vi "trial 2.vi"() -> ()   [LabVIEW 2013]
panel:
  in  "Contours":T1(array[cluster])
  in  "Global Rectangle":i32[](array[numeric])
  in  "ROI Descriptor":T2 {"Contours"."Type" items=["No Selection", "Point", "Line", "Rectangle", "Oval", "Polygon", "Freehand Region", "Annulus", "Unused2", "Unused3", "Broken Line", "Freehand Line", "Rotated Rectangle"]}
  in  "Play":bool
  in  "stop":bool
  in  "Pause":bool
  out "Image 3":T3(plugin-control)
  in  "AVI File Path":path
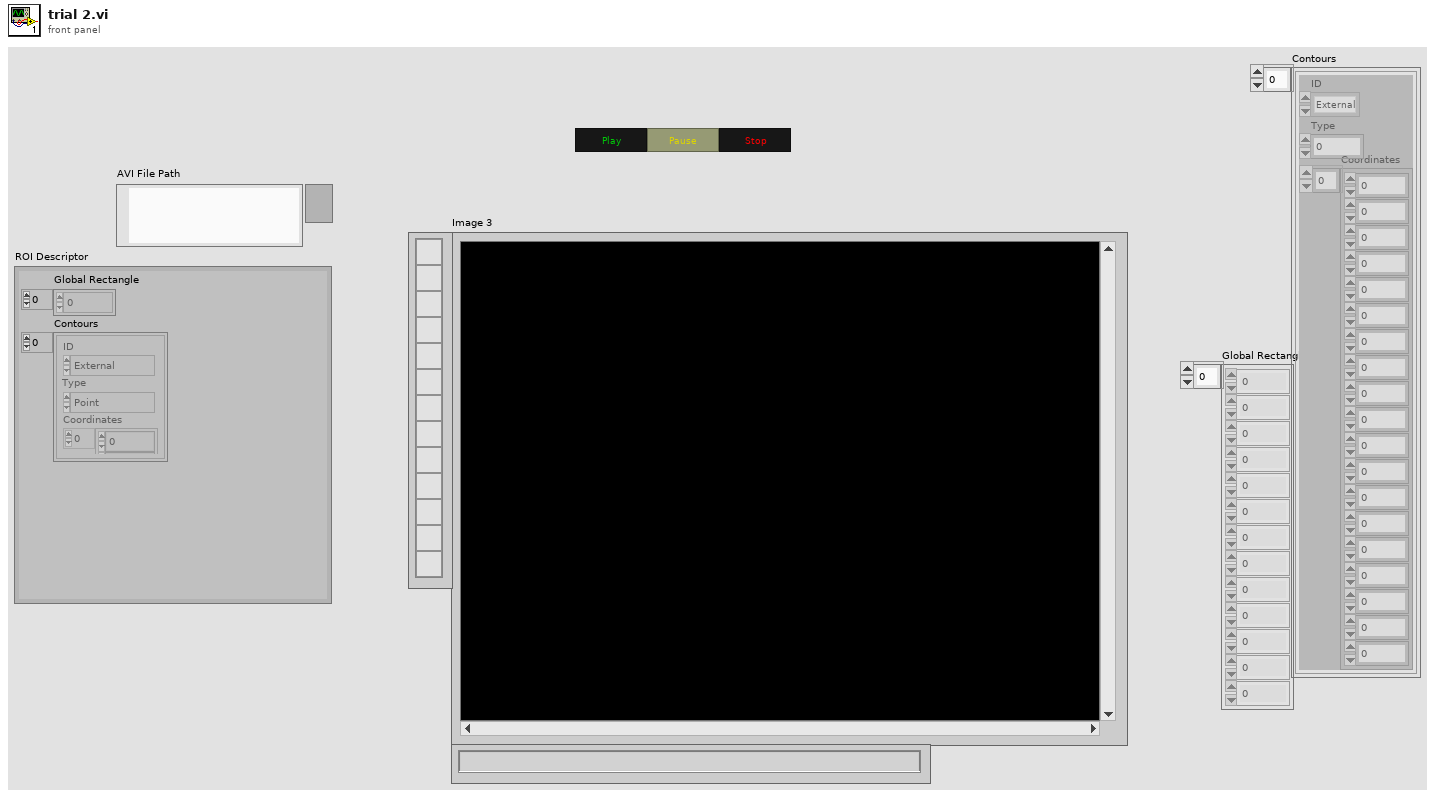
[diagram p1: front panel]
types:
  T1 = cluster{"ID":enum32{"External", "Internal"}, "Type":u32, "Coordinates":i32[]}[]
  T2 = typedef "ROI Descriptor" = cluster{"Global Rectangle":i32[], "Contours":cluster{"ID":enum32{"External", "Internal"}, "Type":u32, "Coordinates":i32[]}[]}
  T3 = typedef "IMAQ Image.ctl" = refnum<image>
  T4 = typedef "Image Type" = u32
  T5 = typedef "AviRefnum.ctl" = refnum<k1>
  T6 = typedef "eventvkey.ctl" = enum16{"ASCII", "Enter", "Return", "Shift", "Ctrl", "Alt", "Cmd", "Opt", "Caps", "NumLock", "Clear", "Break", "Up", "Down", "Left", "Right", "Insert", "Delete", "Home", "End", "PageUp", "PageDown", "Escape", "Help", "Pause", "ScrollLock", "F1", "F2", "F3", "F4", "F5", "F6", "F7", "F8", "F9", "F10", "F11", "F12", "F13", "F14", "F15", "F16", "F17", "F18", "F19", "F20", "F21", "F22", "F23", "F24", "Play", "VolumeUp", "VolumeDown", "Mute", "Two Byte Char"}
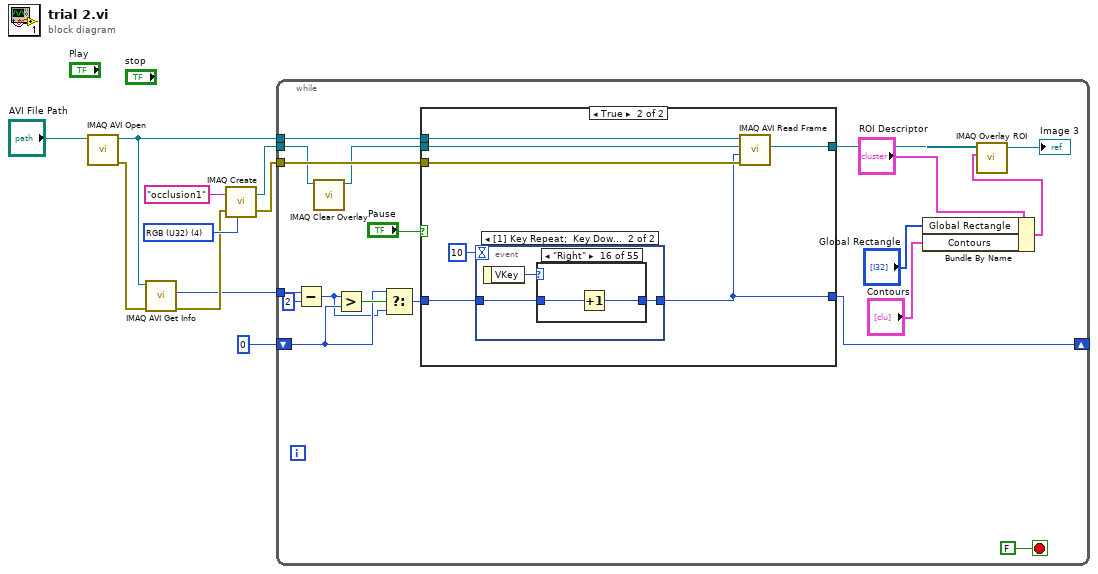
[diagram p0: block diagram]
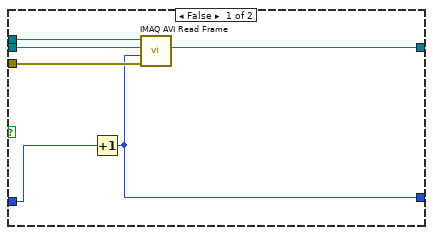
[diagram p2: hidden frame]
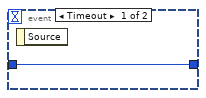
[diagram p3: hidden frame]
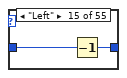
[diagram p18: hidden frame]
diagram:
  w8 = T4 4 items=["Grayscale (U8)", "Grayscale (I16)", "Grayscale (SGL)", "Complex (CSG)", "RGB (U32)", "HSL (U32)", "RGB (U64)", "Grayscale (U16)"] ("Image Type")
  n1 = call "IMAQ AVI Open"("AVI Path"="AVI File Path") -> ("error out"=w4:errorcluster, "Avi Refnum"=w5:T5)  [unwired: 9 in]
  n2 = call "IMAQ AVI Get Info"("error in (no error)"=w4, "Avi Refnum"=w5) -> ("error out"=w3:errorcluster, "Number of Frames"=w2:u32)  [unwired: 5 in, 3 out]
  n3 = call "IMAQ Create"("Image Name"="occlusion1", "Image Type"=w8, "error in (no error)"=w3) -> ("New Image"=w7:T3, "error out"=w6:errorcluster)  [unwired: 2 in]
  n4 = while {
    tunnel: w5 -> [w28]
    tunnel: w7 -> [w12]
    tunnel: w6 -> [w27]
    tunnel: w2 -> [w22]
    shift-right: [w19] -> _
    shift-left: 0 -> [w23]
    stop <- FALSE stop-if-true
    n5 = Subtract(x=w22, y=u32 2) -> (x-y=w20:u32)
    n6 = call "IMAQ Clear Overlay"("Image"=w12) -> ("Image Out"=w11:T3)  [unwired: 9 in, 1 out]
    n7 = Greater?(x=w20, y=w23) -> (0:w25:bool)
    n8 = Select(t=w23, s=w25, f=w20) -> (s? t:f=w24:u32)
    n9 = case shown="True" "Pause" {
      tunnel: w11 -> [w35 w39]
      tunnel: w28 -> [w34 w40]
      tunnel: w27 -> [w33 w38]
      tunnel: w24 -> [w31 w41]
      tunnel: [w32 w37] -> w17
      tunnel: [w30 w36] -> w19
      frame False {
        n10 = Increment(x=w31) -> (x+1=w30:u32)
        n11 = call "IMAQ AVI Read Frame"("error in (no error)"=w33, "Frame Number"=w30, "Image"=w35, "Avi Refnum"=w34) -> ("Image Out"=w32:T3)  [unwired: 4 in, 3 out]
      }
      frame True {
        n12 = event shown="[1] Key Repeat;  Key Down" {
          selector: _ -> [_ _]
          dyn-events: _ -> [_ _]
          timeout: 10 -> [_ _]
          tunnel: w41 -> [w43 w45]
          tunnel: [w43 w44] -> w36
          event Timeout {
            n13 = event-data() -> ()  [unwired: 1 in, 1 out]
          }
          event Key Repeat; Key Down {
            n14 = event-data() -> ("VKey"=w46:T6)  [unwired: 1 in]
            n15 = case shown="\"Right\"" w46 {
              tunnel: w45 -> [w47 w48 w49 w50 w51 w52 w53 w54 w55 w56 w57 w58 w59 w60 w62 w64 w65 w66 w67 w68 w69 w70 w71 w72 w73 w74 w75 w76 w77 w78 w79 w80 w81 w82 w83 w84 w85 w86 w87 w88 w89 w90 w91 w92 w93 w94 w95 w96 w97 w98 w99 w100 w101 w102 w103]
              tunnel: [w47 w48 w49 w50 w51 w52 w53 w54 w55 w56 w57 w58 w59 w60 w61 w63 w65 w66 w67 w68 w69 w70 w71 w72 w73 w74 w75 w76 w77 w78 w79 w80 w81 w82 w83 w84 w85 w86 w87 w88 w89 w90 w91 w92 w93 w94 w95 w96 w97 w98 w99 w100 w101 w102 w103] -> w44
              frame "ASCII", Default {
              }
              frame "Enter" {
              }
              frame "Return" {
              }
              frame "Shift" {
              }
              frame "Ctrl" {
              }
              frame "Alt" {
              }
              frame "Cmd" {
              }
              frame "Opt" {
              }
              frame "Caps" {
              }
              frame "NumLock" {
              }
              frame "Clear" {
              }
              frame "Break" {
              }
              frame "Up" {
              }
              frame "Down" {
              }
              frame "Left" {
                n16 = Decrement(x=w62) -> (x-1=w61:u32)
              }
              frame "Right" {
                n17 = Increment(x=w64) -> (x+1=w63:u32)
              }
              frame "Insert" {
              }
              frame "Delete" {
              }
              frame "Home" {
              }
              frame "End" {
              }
              frame "PageUp" {
              }
              frame "PageDown" {
              }
              frame "Escape" {
              }
              frame "Help" {
              }
              frame "Pause" {
              }
              frame "ScrollLock" {
              }
              frame "F1" {
              }
              frame "F2" {
              }
              frame "F3" {
              }
              frame "F4" {
              }
              frame "F5" {
              }
              frame "F6" {
              }
              frame "F7" {
              }
              frame "F8" {
              }
              frame "F9" {
              }
              frame "F10" {
              }
              frame "F11" {
              }
              frame "F12" {
              }
              frame "F13" {
              }
              frame "F14" {
              }
              frame "F15" {
              }
              frame "F16" {
              }
              frame "F17" {
              }
              frame "F18" {
              }
              frame "F19" {
              }
              frame "F20" {
              }
              frame "F21" {
              }
              frame "F22" {
              }
              frame "F23" {
              }
              frame "F24" {
              }
              frame "Play" {
              }
              frame "VolumeUp" {
              }
              frame "VolumeDown" {
              }
              frame "Mute" {
              }
              frame "Two Byte Char" {
              }
            }
          }
        }
        n18 = call "IMAQ AVI Read Frame"("error in (no error)"=w38, "Frame Number"=w36, "Image"=w39, "Avi Refnum"=w40) -> ("Image Out"=w37:T3)  [unwired: 4 in, 3 out]
      }
    }
    n19 = Bundle By Name(cluster="ROI Descriptor", "Global Rectangle"="Global Rectangle", "Contours"="Contours") -> (w15:T2)
    n20 = call "IMAQ Overlay ROI"("ROI Descriptor"=w15, "Image"=w17) -> ("Image Out"=→"Image 3":T3)  [unwired: 8 in, 1 out]
  }
